vi "Windows Main-forDOG.vi"() -> ()   [LabVIEW 2016]
uses:
  <resource>/objmgr/ni.dex.rc
panel:
  in  "停止应用程序 15":bool
  out "Array 14":i32[][](array[numeric])
  in  "停止应用程序 14":bool
  out "Array 13":i32[][](array[numeric])
  in  "停止应用程序 13":bool
  out "Array 12":i32[][](array[numeric])
  in  "停止应用程序 12":bool
  out "Array 11":i32[][](array[numeric])
  in  "停止应用程序 11":bool
  out "Array 10":i32[][](array[numeric])
  in  "停止应用程序 10":bool
  out "Array 9":i32[][](array[numeric])
  in  "停止应用程序 9":bool
  out "Gaussian2-4":T1(plugin-control)
  out "Array 8":i32[][](array[numeric])
  in  "停止应用程序 8":bool
  out "Gaussian2-3":T1(plugin-control)
  out "Array 7":i32[][](array[numeric])
  in  "停止应用程序 7":bool
  out "Gaussian2-2":T1(plugin-control)
  out "Array 6":i32[][](array[numeric])
  in  "停止应用程序 6":bool
  out "Gaussian2-1":T1(plugin-control)
  out "Array 5":i32[][](array[numeric])
  in  "停止应用程序 5":bool
  out "Gaussian1-4":T1(plugin-control)
  out "Array 4":i32[][](array[numeric])
  in  "停止应用程序 4":bool
  out "Gaussian1-3":T1(plugin-control)
  out "Array 3":i32[][](array[numeric])
  in  "停止应用程序 3":bool
  out "Gaussian1-2":T1(plugin-control)
  out "Array 2":i32[][](array[numeric])
  out "error out 2":errorcluster
  in  "停止应用程序 2":bool
  out "OriImage":T1(plugin-control)
  out "Array":i32[][](array[numeric])
  out "Numeric":i32
  in  "终端IP地址":string
  out "error out":errorcluster
  in  "停止应用程序":bool
  out "Gaussian1-1":T1(plugin-control)
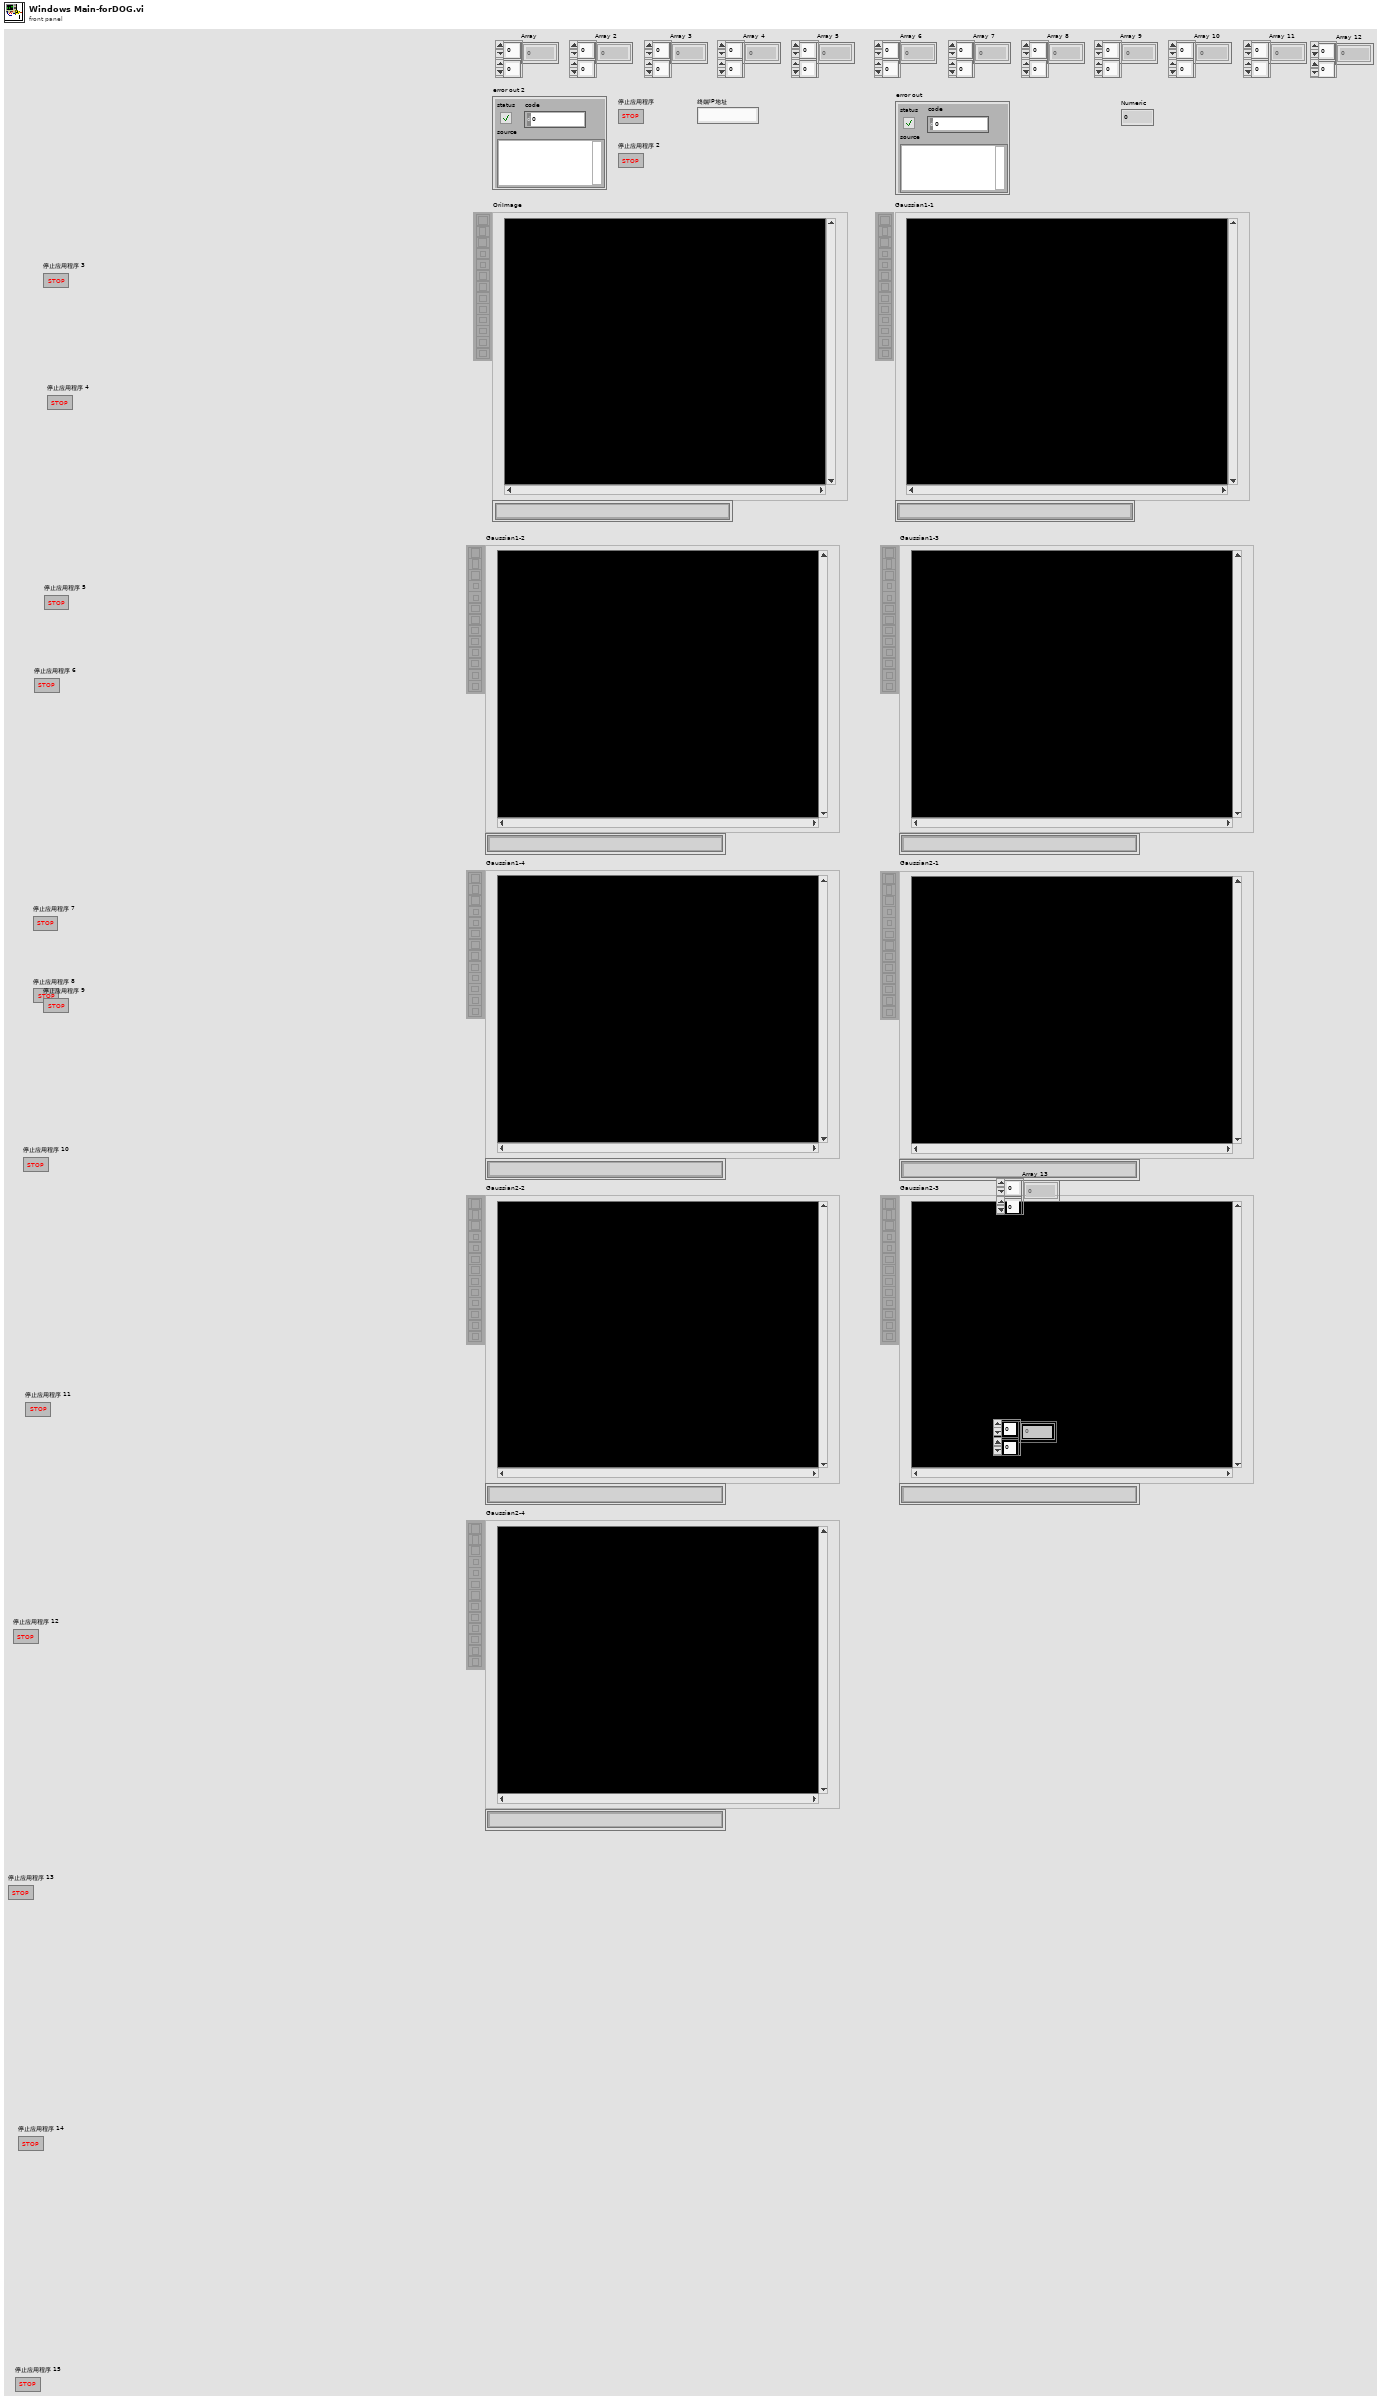
[diagram p1: front panel]
types:
  T1 = typedef "IMAQ Image.ctl" = refnum<image>
  T2 = typedef "Image Type" = u32
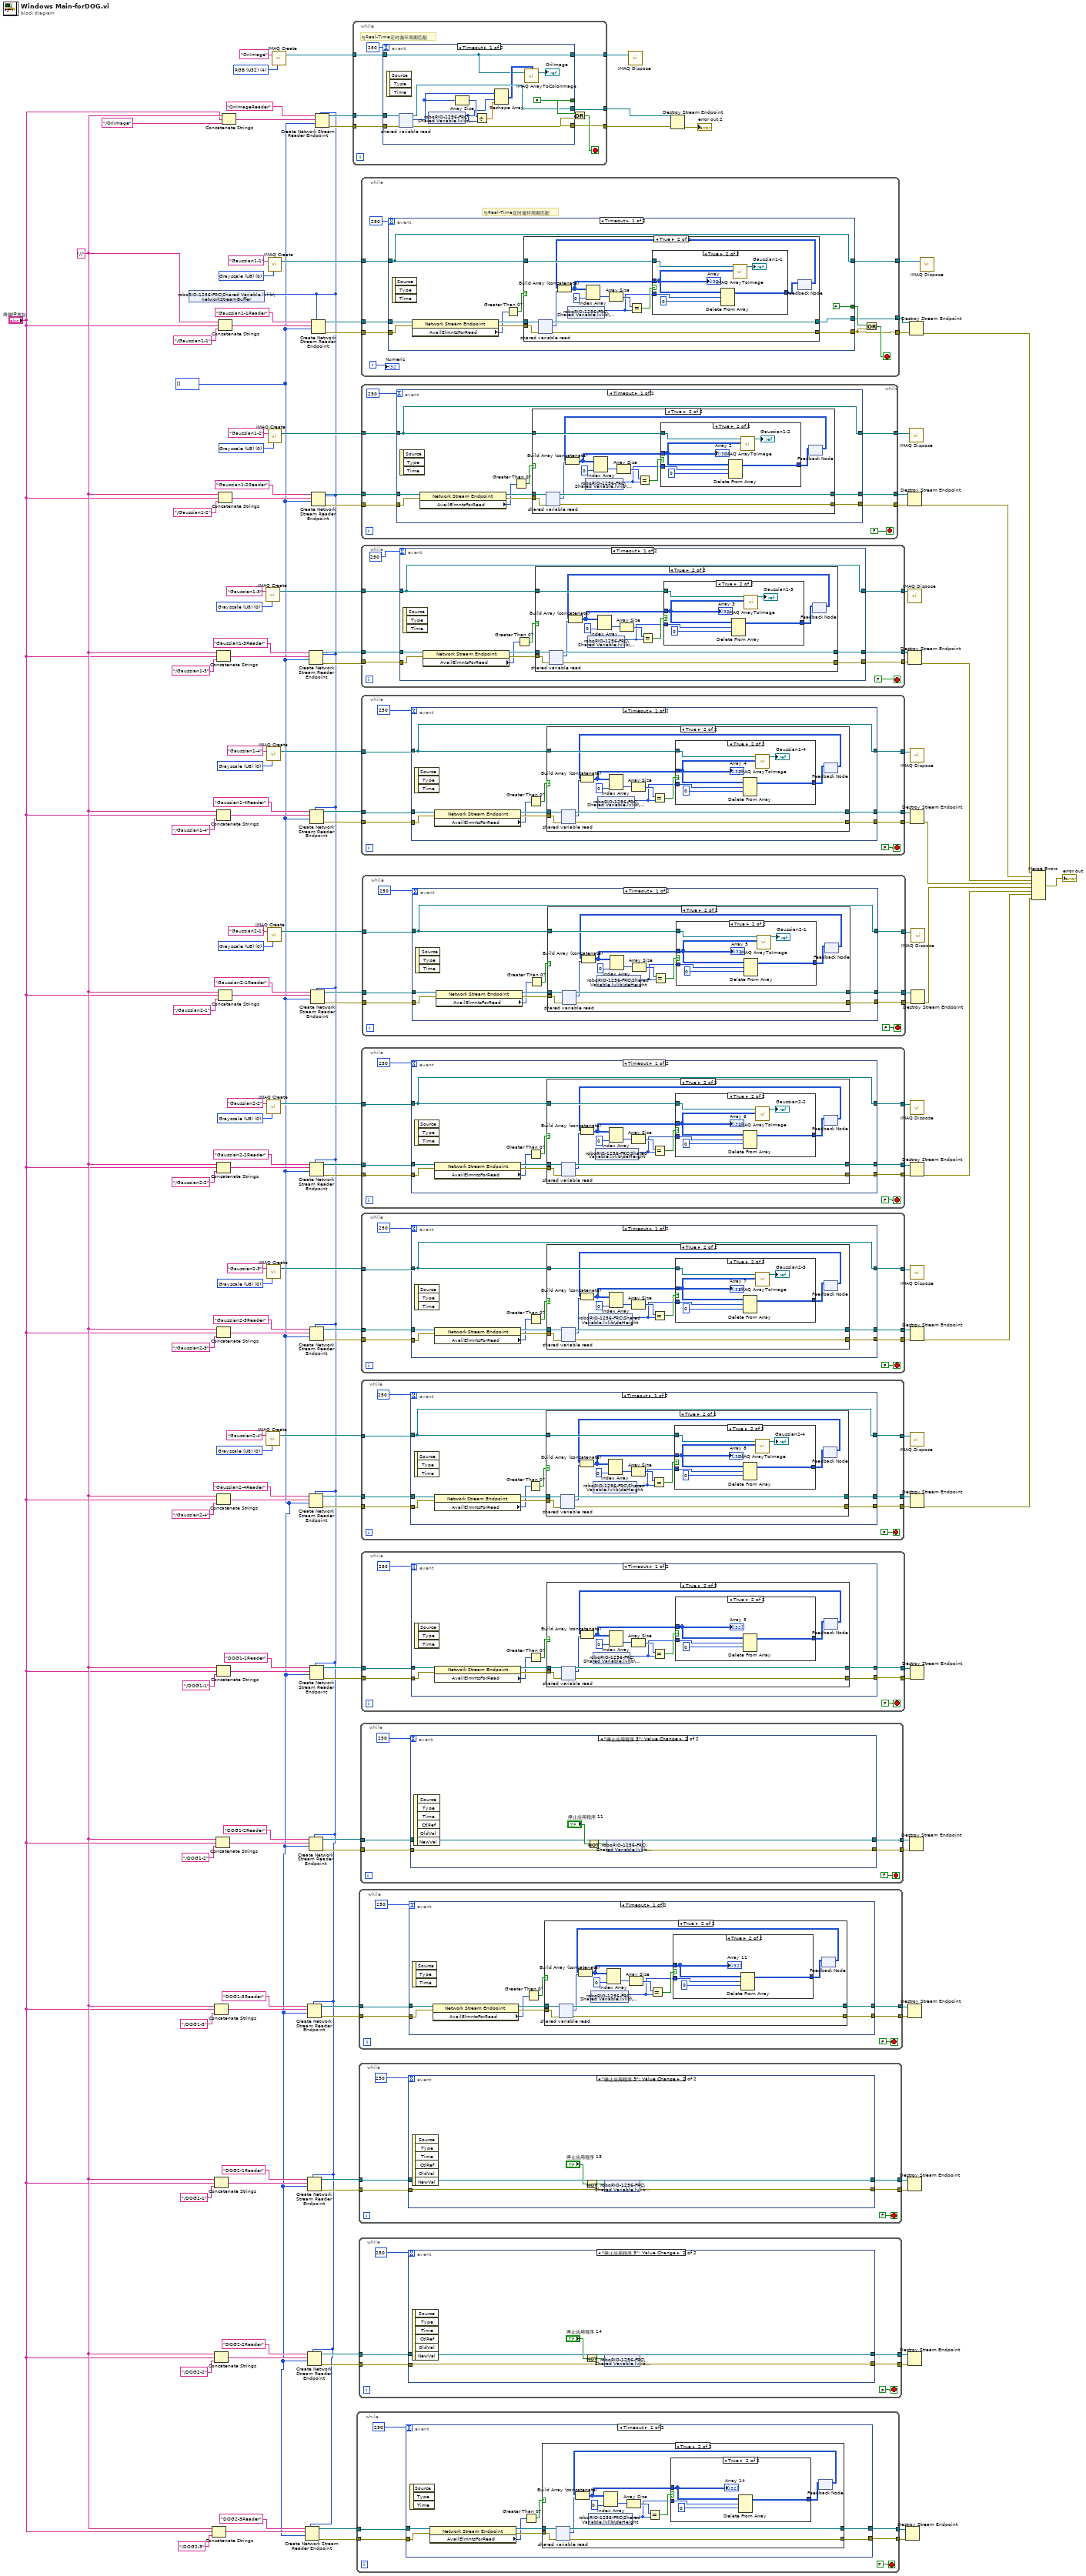
[diagram p0: block diagram]
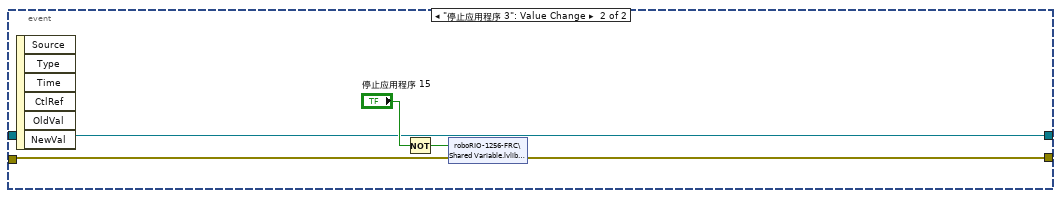
[diagram p4: hidden frame]
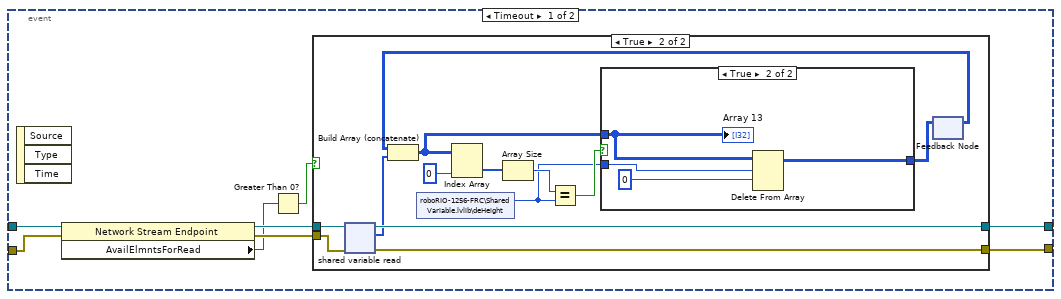
[diagram p5: hidden frame]
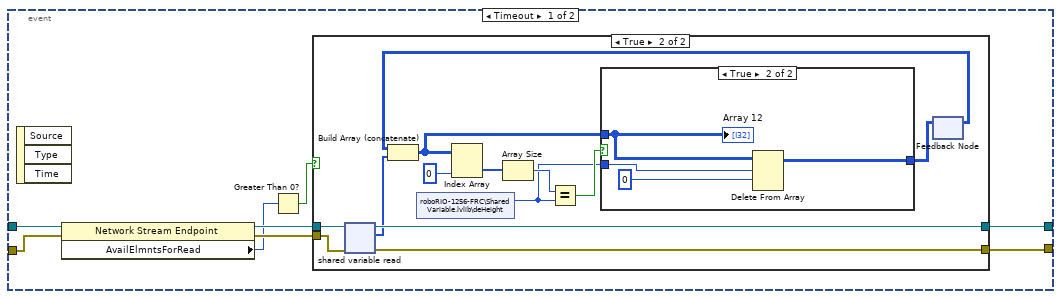
[diagram p8: hidden frame]
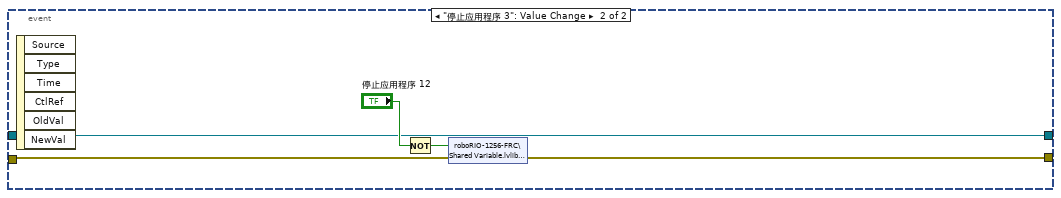
[diagram p13: hidden frame]
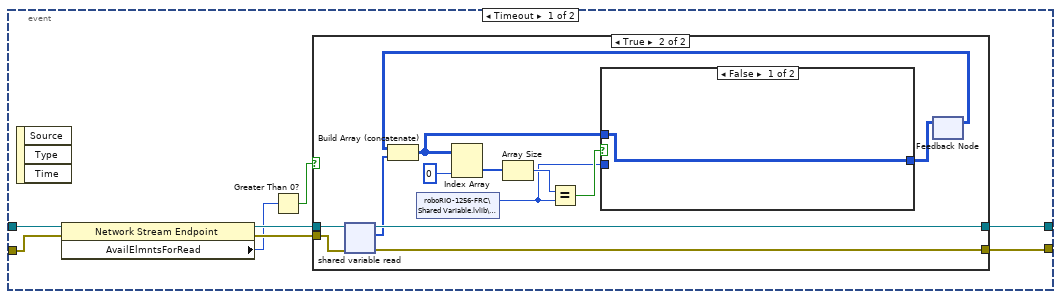
[diagram p14: hidden frame]
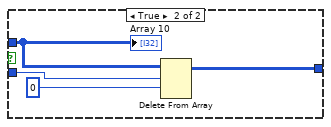
[diagram p16: hidden frame]
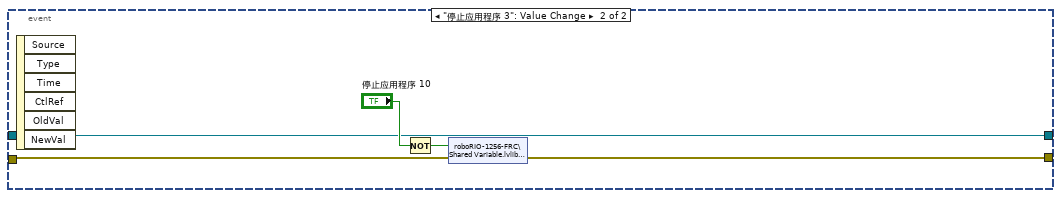
[diagram p19: hidden frame]
diagram:
  w60 = T2 0 items=["Grayscale (U8)", "Grayscale (I16)", "Grayscale (SGL)", "Complex (CSG)", "RGB (U32)", "HSL (U32)", "RGB (U64)", "Grayscale (U16)"] ("Image Type")
  w61 = T2 0 items=["Grayscale (U8)", "Grayscale (I16)", "Grayscale (SGL)", "Complex (CSG)", "RGB (U32)", "HSL (U32)", "RGB (U64)", "Grayscale (U16)"] ("Image Type")
  w82 = T2 0 items=["Grayscale (U8)", "Grayscale (I16)", "Grayscale (SGL)", "Complex (CSG)", "RGB (U32)", "HSL (U32)", "RGB (U64)", "Grayscale (U16)"] ("Image Type")
  w84 = T2 0 items=["Grayscale (U8)", "Grayscale (I16)", "Grayscale (SGL)", "Complex (CSG)", "RGB (U32)", "HSL (U32)", "RGB (U64)", "Grayscale (U16)"] ("Image Type")
  w118 = T2 0 items=["Grayscale (U8)", "Grayscale (I16)", "Grayscale (SGL)", "Complex (CSG)", "RGB (U32)", "HSL (U32)", "RGB (U64)", "Grayscale (U16)"] ("Image Type")
  w123 = T2 0 items=["Grayscale (U8)", "Grayscale (I16)", "Grayscale (SGL)", "Complex (CSG)", "RGB (U32)", "HSL (U32)", "RGB (U64)", "Grayscale (U16)"] ("Image Type")
  w124 = T2 0 items=["Grayscale (U8)", "Grayscale (I16)", "Grayscale (SGL)", "Complex (CSG)", "RGB (U32)", "HSL (U32)", "RGB (U64)", "Grayscale (U16)"] ("Image Type")
  w136 = T2 4 items=["Grayscale (U8)", "Grayscale (I16)", "Grayscale (SGL)", "Complex (CSG)", "RGB (U32)", "HSL (U32)", "RGB (U64)", "Grayscale (U16)"] ("Image Type")
  w129 = T2 0 items=["Grayscale (U8)", "Grayscale (I16)", "Grayscale (SGL)", "Complex (CSG)", "RGB (U32)", "HSL (U32)", "RGB (U64)", "Grayscale (U16)"] ("Image Type")
  w3 = i32[] []
  w2 = "//" ("string")
  n1 = shared-variable "roboRIO-1256-FRC\\Shared Variable.lvlib\\networkStreamBuffer"() -> (w4:i8)  [unwired: 1 in, 1 out]
  n2 = Concatenate Strings(w2, "终端IP地址", "/DOG2-3" ("string")) -> (w9:string)
  n3 = Concatenate Strings(w2, "终端IP地址", "/DOG2-1" ("string")) -> (w23:string)
  n4 = Concatenate Strings(w2, "终端IP地址", "/DOG2-2" ("string")) -> (w14:string)
  n5 = Concatenate Strings(w2, "终端IP地址", "/DOG1-3" ("string")) -> (w28:string)
  n6 = Concatenate Strings(w2, "终端IP地址", "/DOG1-2" ("string")) -> (w37:string)
  n7 = Concatenate Strings(w2, "终端IP地址", "/Gaussian1-3" ("string")) -> (w127:string)
  n8 = Concatenate Strings(w2, "终端IP地址", "/Gaussian2-4" ("string")) -> (w57:string)
  n9 = Concatenate Strings(w2, "终端IP地址", "/Gaussian1-4" ("string")) -> (w115:string)
  n10 = Concatenate Strings(w2, "终端IP地址", "/Gaussian2-2" ("string")) -> (w79:string)
  n11 = Concatenate Strings(w2, "终端IP地址", "/Gaussian2-3" ("string")) -> (w64:string)
  n12 = Concatenate Strings(w2, "终端IP地址", "/DOG1-1" ("string")) -> (w42:string)
  n13 = Concatenate Strings(w2, "终端IP地址", "/Gaussian2-1" ("string")) -> (w87:string)
  n14 = Concatenate Strings(w2, "终端IP地址", "/Gaussian1-1" ("string")) -> (w152:string)
  n15 = Concatenate Strings(w2, "终端IP地址", "/Gaussian1-2" ("string")) -> (w131:string)
  n16 = Concatenate Strings(w2, "终端IP地址", "/OriImage" ("string")) -> (w142:string)
  n17 = call "IMAQ Create"("Image Name"="Gaussian1-3", "Image Type"=w123) -> ("New Image"=w106:T1)  [unwired: 3 in, 1 out]
  n18 = call "IMAQ Create"("Image Name"="Gaussian2-4", "Image Type"=w60) -> ("New Image"=w55:T1)  [unwired: 3 in, 1 out]
  n19 = call "IMAQ Create"("Image Name"="Gaussian1-4", "Image Type"=w118) -> ("New Image"=w112:T1)  [unwired: 3 in, 1 out]
  n20 = call "IMAQ Create"("Image Name"="Gaussian2-2", "Image Type"=w82) -> ("New Image"=w77:T1)  [unwired: 3 in, 1 out]
  n21 = call "IMAQ Create"("Image Name"="Gaussian2-3", "Image Type"=w61) -> ("New Image"=w66:T1)  [unwired: 3 in, 1 out]
  n22 = call "IMAQ Create"("Image Name"="Gaussian2-1", "Image Type"=w84) -> ("New Image"=w89:T1)  [unwired: 3 in, 1 out]
  n23 = call "IMAQ Create"("Image Name"="Gaussian1-1", "Image Type"=w129) -> ("New Image"=w148:T1)  [unwired: 3 in, 1 out]
  n24 = call "IMAQ Create"("Image Name"="Gaussian1-2", "Image Type"=w124) -> ("New Image"=w98:T1)  [unwired: 3 in, 1 out]
  n25 = call "IMAQ Create"("Image Name"="OriImage", "Image Type"=w136) -> ("New Image"=w135:T1)  [unwired: 3 in, 1 out]
  n26 = Create Network Stream Reader Endpoint(7:w4, 9:w3, 10:w9, 11:"DOG2-3Reader" ("reader name")) -> (0:w7:errorcluster, 3:w8:refnum<k21>)  [unwired: 3 in]
  n27 = Create Network Stream Reader Endpoint(7:w4, 9:w3, 10:w23, 11:"DOG2-1Reader" ("reader name")) -> (0:w21:errorcluster, 3:w22:refnum<k21>)  [unwired: 3 in]
  n28 = Create Network Stream Reader Endpoint(7:w4, 9:w3, 10:w14, 11:"DOG2-2Reader" ("reader name")) -> (0:w16:errorcluster, 3:w15:refnum<k21>)  [unwired: 3 in]
  n29 = Create Network Stream Reader Endpoint(7:w4, 9:w3, 10:w28, 11:"DOG1-3Reader" ("reader name")) -> (0:w30:errorcluster, 3:w29:refnum<k21>)  [unwired: 3 in]
  n30 = Create Network Stream Reader Endpoint(7:w4, 9:w3, 10:w37, 11:"DOG1-2Reader" ("reader name")) -> (0:w35:errorcluster, 3:w36:refnum<k21>)  [unwired: 3 in]
  n31 = Create Network Stream Reader Endpoint(7:w4, 9:w3, 10:w127, 11:"Gaussian1-3Reader" ("reader name")) -> (0:w104:errorcluster, 3:w105:refnum<k21>)  [unwired: 3 in]
  n32 = Create Network Stream Reader Endpoint(7:w4, 9:w3, 10:w57, 11:"Gaussian2-4Reader" ("reader name")) -> (0:w53:errorcluster, 3:w54:refnum<k21>)  [unwired: 3 in]
  n33 = Create Network Stream Reader Endpoint(7:w4, 9:w3, 10:w115, 11:"Gaussian1-4Reader" ("reader name")) -> (0:w110:errorcluster, 3:w111:refnum<k21>)  [unwired: 3 in]
  n34 = Create Network Stream Reader Endpoint(7:w4, 9:w3, 10:w79, 11:"Gaussian2-2Reader" ("reader name")) -> (0:w75:errorcluster, 3:w76:refnum<k21>)  [unwired: 3 in]
  n35 = Create Network Stream Reader Endpoint(7:w4, 9:w3, 10:w64, 11:"Gaussian2-3Reader" ("reader name")) -> (0:w68:errorcluster, 3:w67:refnum<k21>)  [unwired: 3 in]
  n36 = Create Network Stream Reader Endpoint(7:w4, 9:w3, 10:w42, 11:"DOG1-1Reader" ("reader name")) -> (0:w44:errorcluster, 3:w43:refnum<k21>)  [unwired: 3 in]
  n37 = Create Network Stream Reader Endpoint(7:w4, 9:w3, 10:w87, 11:"Gaussian2-1Reader" ("reader name")) -> (0:w91:errorcluster, 3:w90:refnum<k21>)  [unwired: 3 in]
  n38 = Create Network Stream Reader Endpoint(7:w4, 9:w3, 10:w152, 11:"Gaussian1-1Reader" ("reader name")) -> (0:w155:errorcluster, 3:w146:refnum<k21>)  [unwired: 3 in]
  n39 = Create Network Stream Reader Endpoint(7:w4, 9:w3, 10:w131, 11:"Gaussian1-2Reader" ("reader name")) -> (0:w99:errorcluster, 3:w100:refnum<k21>)  [unwired: 3 in]
  n40 = Create Network Stream Reader Endpoint(7:w4, 9:w3, 10:w142, 11:"OriImageReader" ("reader name")) -> (0:w145:errorcluster, 3:w140:refnum<k21>)  [unwired: 3 in]
  n41 = while {
    tunnel: w140 -> [w159]
    tunnel: [w158] -> w139
    tunnel: w135 -> [w157]
    tunnel: [w156] -> w134
    tunnel: w145 -> [w161]
    tunnel: [w160] -> w141
    stop <- w162 stop-if-true
    # "与Real-Time定时循环周期匹配"
    n42 = event shown="[0] Timeout" {
      selector: _ -> [_ _]
      dyn-events: _ -> [_ _]
      timeout: 250 -> [_ _]
      tunnel: [FALSE ("停止应用程序") "停止应用程序 2"] -> w163
      tunnel: w161 -> [w176 w180]
      tunnel: [w175 w179] -> w160
      tunnel: w159 -> [w174 w177]
      tunnel: [w173 w177] -> w158
      tunnel: w157 -> [w166 w178]
      tunnel: [w166 w178] -> w156
      event Timeout {
        n43 = event-data() -> ()  [unwired: 1 in, 3 out]
        n44 = shared-variable-read(w174, w176) -> (w173:refnum<k21>, w175:errorcluster, w169:i32[])  [unwired: 1 in, 1 out]
        n45 = shared-variable "roboRIO-1256-FRC\\Shared Variable.lvlib\\Height"() -> (w165:u16)  [unwired: 1 in, 1 out]
        n46 = Array Size(array=w169) -> (size(s)=w171:i32)
        n47 = Divide(x=w171, y=w165) -> (x/y=w170:dbl)
        n48 = Reshape Array(w169, w165, w170) -> (w168:i32[][])
        n49 = call "IMAQ ArrayToColorImage"("Image Pixels (U32)"=w168, "Image"=w166) -> ("Image Out"=→"OriImage":T1)  [unwired: 3 in, 1 out]
      }
      event "停止应用程序 2": Value Change {
        n50 = event-data() -> ()  [unwired: 1 in, 6 out]
        n51 = Not(x="停止应用程序 2") -> (.not. x?=w181:bool)
        n52 = shared-variable "roboRIO-1256-FRC\\Shared Variable.lvlib\\Active"(w181, error in=w180) -> (error out=w179:errorcluster)
      }
    }
    n53 = Or(x=w163, y=w160) -> (x .or. y?=w162:bool)
  }
  n54 = while {
    tunnel: w8 -> [w188]
    tunnel: [w185] -> w5
    tunnel: w7 -> [w187]
    tunnel: [w186] -> w6
    stop <- FALSE stop-if-true
    n55 = event shown="[0] Timeout" {
      selector: _ -> [_ _]
      dyn-events: _ -> [_ _]
      timeout: 250 -> [_ _]
      tunnel: w187 -> [w194 w219]
      tunnel: [w196 w218] -> w186
      tunnel: w188 -> [w193 w217]
      tunnel: [w195 w217] -> w185
      event Timeout {
        n56 = event-data() -> ()  [unwired: 1 in, 3 out]
        n57 = property class="Network Stream Endpoint"(reference=w193, error in=w194) -> (reference out=w191:refnum<k21>, error out=w192:errorcluster, "AvailElmntsForRead"=w190:i32)
        n58 = Greater Than 0?(x=w190) -> (x > 0?=w189:bool)
        n59 = case shown="True" w189 {
          tunnel: [w197 w211] -> w196
          tunnel: [w198 w210] -> w195
          tunnel: w192 -> [w197 w205]
          tunnel: w191 -> [w198 w204]
          frame False {
          }
          frame True {
            n60 = shared-variable-read(w204, w205) -> (w210:refnum<k21>, w211:errorcluster, w202:i32[])  [unwired: 1 in, 1 out]
            n61 = shared-variable "roboRIO-1256-FRC\\Shared Variable.lvlib\\deHeight"() -> (w199:u16)  [unwired: 1 in, 1 out]
            n62 = feedback #1() -> (w200:i32[][])  [unwired: 1 in]
            n63 = Build Array (concatenate)(w200, w202) -> (w203:i32[][])
            n64 = Index Array(array=w203, index (col)=0 ("disabled index (col)")) -> (element=w208:i32[])  [unwired: 1 in]
            n65 = Array Size(array=w208) -> (size(s)=w207:i32)
            n66 = Equal?(x=w207, y=w199) -> (x = y?=w206:bool)
            n67 = case shown="True" w206 {
              tunnel: w203 -> [w212 w213]
              tunnel: [w212 w214] -> w201
              tunnel: w199 -> [_ w216]
              frame False {
              }
              frame True {
                n68 = Delete From Array(array=w213, length=w216, index (row)=0) -> (array with subset deleted=w214:i32[][])  [unwired: 1 in, 1 out]
                "Array 14" <- w213
              }
            }
            n69 = feedback-in #1(w201) -> ()
          }
        }
      }
      event "停止应用程序 3": Value Change {
        n70 = event-data() -> ()  [unwired: 1 in, 6 out]
        n71 = Not(x="停止应用程序 15") -> (.not. x?=w220:bool)
        n72 = shared-variable "roboRIO-1256-FRC\\Shared Variable.lvlib\\Active"(w220, error in=w219) -> (error out=w218:errorcluster)
      }
    }
  }
  n73 = while {
    tunnel: w22 -> [w227]
    tunnel: [w224] -> w19
    tunnel: w21 -> [w226]
    tunnel: [w225] -> w20
    stop <- FALSE stop-if-true
    n74 = event shown="[1] \"停止应用程序 3\": Value Change" {
      selector: _ -> [_ _]
      dyn-events: _ -> [_ _]
      timeout: 250 -> [_ _]
      tunnel: w226 -> [w233 w258]
      tunnel: [w235 w257] -> w225
      tunnel: w227 -> [w232 w256]
      tunnel: [w234 w256] -> w224
      event Timeout {
        n75 = event-data() -> ()  [unwired: 1 in, 3 out]
        n76 = property class="Network Stream Endpoint"(reference=w232, error in=w233) -> (reference out=w230:refnum<k21>, error out=w231:errorcluster, "AvailElmntsForRead"=w229:i32)
        n77 = Greater Than 0?(x=w229) -> (x > 0?=w228:bool)
        n78 = case shown="True" w228 {
          tunnel: [w236 w250] -> w235
          tunnel: [w237 w249] -> w234
          tunnel: w231 -> [w236 w244]
          tunnel: w230 -> [w237 w243]
          frame False {
          }
          frame True {
            n79 = shared-variable-read(w243, w244) -> (w249:refnum<k21>, w250:errorcluster, w241:i32[])  [unwired: 1 in, 1 out]
            n80 = shared-variable "roboRIO-1256-FRC\\Shared Variable.lvlib\\deHeight"() -> (w238:u16)  [unwired: 1 in, 1 out]
            n81 = feedback #2() -> (w239:i32[][])  [unwired: 1 in]
            n82 = Build Array (concatenate)(w239, w241) -> (w242:i32[][])
            n83 = Index Array(array=w242, index (col)=0 ("disabled index (col)")) -> (element=w247:i32[])  [unwired: 1 in]
            n84 = Array Size(array=w247) -> (size(s)=w246:i32)
            n85 = Equal?(x=w246, y=w238) -> (x = y?=w245:bool)
            n86 = case shown="True" w245 {
              tunnel: w242 -> [w251 w252]
              tunnel: [w251 w253] -> w240
              tunnel: w238 -> [_ w255]
              frame False {
              }
              frame True {
                n87 = Delete From Array(array=w252, length=w255, index (row)=0) -> (array with subset deleted=w253:i32[][])  [unwired: 1 in, 1 out]
                "Array 12" <- w252
              }
            }
            n88 = feedback-in #2(w240) -> ()
          }
        }
      }
      event "停止应用程序 3": Value Change {
        n89 = event-data() -> ()  [unwired: 1 in, 6 out]
        n90 = Not(x="停止应用程序 13") -> (.not. x?=w259:bool)
        n91 = shared-variable "roboRIO-1256-FRC\\Shared Variable.lvlib\\Active"(w259, error in=w258) -> (error out=w257:errorcluster)
      }
    }
  }
  n92 = while {
    tunnel: w15 -> [w266]
    tunnel: [w263] -> w18
    tunnel: w16 -> [w265]
    tunnel: [w264] -> w17
    stop <- FALSE stop-if-true
    n93 = event shown="[1] \"停止应用程序 3\": Value Change" {
      selector: _ -> [_ _]
      dyn-events: _ -> [_ _]
      timeout: 250 -> [_ _]
      tunnel: w265 -> [w272 w297]
      tunnel: [w274 w296] -> w264
      tunnel: w266 -> [w271 w295]
      tunnel: [w273 w295] -> w263
      event Timeout {
        n94 = event-data() -> ()  [unwired: 1 in, 3 out]
        n95 = property class="Network Stream Endpoint"(reference=w271, error in=w272) -> (reference out=w269:refnum<k21>, error out=w270:errorcluster, "AvailElmntsForRead"=w268:i32)
        n96 = Greater Than 0?(x=w268) -> (x > 0?=w267:bool)
        n97 = case shown="True" w267 {
          tunnel: [w275 w289] -> w274
          tunnel: [w276 w288] -> w273
          tunnel: w270 -> [w275 w283]
          tunnel: w269 -> [w276 w282]
          frame False {
          }
          frame True {
            n98 = shared-variable-read(w282, w283) -> (w288:refnum<k21>, w289:errorcluster, w280:i32[])  [unwired: 1 in, 1 out]
            n99 = shared-variable "roboRIO-1256-FRC\\Shared Variable.lvlib\\deHeight"() -> (w277:u16)  [unwired: 1 in, 1 out]
            n100 = feedback #3() -> (w278:i32[][])  [unwired: 1 in]
            n101 = Build Array (concatenate)(w278, w280) -> (w281:i32[][])
            n102 = Index Array(array=w281, index (col)=0 ("disabled index (col)")) -> (element=w286:i32[])  [unwired: 1 in]
            n103 = Array Size(array=w286) -> (size(s)=w285:i32)
            n104 = Equal?(x=w285, y=w277) -> (x = y?=w284:bool)
            n105 = case shown="True" w284 {
              tunnel: w281 -> [w290 w291]
              tunnel: [w290 w292] -> w279
              tunnel: w277 -> [_ w294]
              frame False {
              }
              frame True {
                n106 = Delete From Array(array=w291, length=w294, index (row)=0) -> (array with subset deleted=w292:i32[][])  [unwired: 1 in, 1 out]
                "Array 13" <- w291
              }
            }
            n107 = feedback-in #3(w279) -> ()
          }
        }
      }
      event "停止应用程序 3": Value Change {
        n108 = event-data() -> ()  [unwired: 1 in, 6 out]
        n109 = Not(x="停止应用程序 14") -> (.not. x?=w298:bool)
        n110 = shared-variable "roboRIO-1256-FRC\\Shared Variable.lvlib\\Active"(w298, error in=w297) -> (error out=w296:errorcluster)
      }
    }
  }
  n111 = while {
    tunnel: w29 -> [w305]
    tunnel: [w302] -> w32
    tunnel: w30 -> [w304]
    tunnel: [w303] -> w31
    stop <- FALSE stop-if-true
    n112 = event shown="[0] Timeout" {
      selector: _ -> [_ _]
      dyn-events: _ -> [_ _]
      timeout: 250 -> [_ _]
      tunnel: w304 -> [w311 w336]
      tunnel: [w313 w335] -> w303
      tunnel: w305 -> [w310 w334]
      tunnel: [w312 w334] -> w302
      event Timeout {
        n113 = event-data() -> ()  [unwired: 1 in, 3 out]
        n114 = property class="Network Stream Endpoint"(reference=w310, error in=w311) -> (reference out=w308:refnum<k21>, error out=w309:errorcluster, "AvailElmntsForRead"=w307:i32)
        n115 = Greater Than 0?(x=w307) -> (x > 0?=w306:bool)
        n116 = case shown="True" w306 {
          tunnel: [w314 w328] -> w313
          tunnel: [w315 w327] -> w312
          tunnel: w309 -> [w314 w322]
          tunnel: w308 -> [w315 w321]
          frame False {
          }
          frame True {
            n117 = shared-variable-read(w321, w322) -> (w327:refnum<k21>, w328:errorcluster, w319:i32[])  [unwired: 1 in, 1 out]
            n118 = shared-variable "roboRIO-1256-FRC\\Shared Variable.lvlib\\Height"() -> (w316:u16)  [unwired: 1 in, 1 out]
            n119 = feedback #4() -> (w317:i32[][])  [unwired: 1 in]
            n120 = Build Array (concatenate)(w317, w319) -> (w320:i32[][])
            n121 = Index Array(array=w320, index (col)=0 ("disabled index (col)")) -> (element=w325:i32[])  [unwired: 1 in]
            n122 = Array Size(array=w325) -> (size(s)=w324:i32)
            n123 = Equal?(x=w324, y=w316) -> (x = y?=w323:bool)
            n124 = case shown="True" w323 {
              tunnel: w320 -> [w329 w330]
              tunnel: [w329 w331] -> w318
              tunnel: w316 -> [_ w333]
              frame False {
              }
              frame True {
                n125 = Delete From Array(array=w330, length=w333, index (row)=0) -> (array with subset deleted=w331:i32[][])  [unwired: 1 in, 1 out]
                "Array 11" <- w330
              }
            }
            n126 = feedback-in #4(w318) -> ()
          }
        }
      }
      event "停止应用程序 3": Value Change {
        n127 = event-data() -> ()  [unwired: 1 in, 6 out]
        n128 = Not(x="停止应用程序 12") -> (.not. x?=w337:bool)
        n129 = shared-variable "roboRIO-1256-FRC\\Shared Variable.lvlib\\Active"(w337, error in=w336) -> (error out=w335:errorcluster)
      }
    }
  }
  n130 = while {
    tunnel: w36 -> [w344]
    tunnel: [w341] -> w33
    tunnel: w35 -> [w343]
    tunnel: [w342] -> w34
    stop <- FALSE stop-if-true
    n131 = event shown="[1] \"停止应用程序 3\": Value Change" {
      selector: _ -> [_ _]
      dyn-events: _ -> [_ _]
      timeout: 250 -> [_ _]
      tunnel: w343 -> [w350 w375]
      tunnel: [w352 w374] -> w342
      tunnel: w344 -> [w349 w373]
      tunnel: [w351 w373] -> w341
      event Timeout {
        n132 = event-data() -> ()  [unwired: 1 in, 3 out]
        n133 = property class="Network Stream Endpoint"(reference=w349, error in=w350) -> (reference out=w347:refnum<k21>, error out=w348:errorcluster, "AvailElmntsForRead"=w346:i32)
        n134 = Greater Than 0?(x=w346) -> (x > 0?=w345:bool)
        n135 = case shown="True" w345 {
          tunnel: [w353 w367] -> w352
          tunnel: [w354 w366] -> w351
          tunnel: w348 -> [w353 w361]
          tunnel: w347 -> [w354 w360]
          frame False {
          }
          frame True {
            n136 = shared-variable-read(w360, w361) -> (w366:refnum<k21>, w367:errorcluster, w358:i32[])  [unwired: 1 in, 1 out]
            n137 = shared-variable "roboRIO-1256-FRC\\Shared Variable.lvlib\\Height"() -> (w355:u16)  [unwired: 1 in, 1 out]
            n138 = feedback #5() -> (w356:i32[][])  [unwired: 1 in]
            n139 = Build Array (concatenate)(w356, w358) -> (w359:i32[][])
            n140 = Index Array(array=w359, index (col)=0 ("disabled index (col)")) -> (element=w364:i32[])  [unwired: 1 in]
            n141 = Array Size(array=w364) -> (size(s)=w363:i32)
            n142 = Equal?(x=w363, y=w355) -> (x = y?=w362:bool)
            n143 = case shown="False" w362 {
              tunnel: w359 -> [w368 w369]
              tunnel: [w368 w370] -> w357
              tunnel: w355 -> [_ w372]
              frame False {
              }
              frame True {
                n144 = Delete From Array(array=w369, length=w372, index (row)=0) -> (array with subset deleted=w370:i32[][])  [unwired: 1 in, 1 out]
                "Array 10" <- w369
              }
            }
            n145 = feedback-in #5(w357) -> ()
          }
        }
      }
      event "停止应用程序 3": Value Change {
        n146 = event-data() -> ()  [unwired: 1 in, 6 out]
        n147 = Not(x="停止应用程序 11") -> (.not. x?=w376:bool)
        n148 = shared-variable "roboRIO-1256-FRC\\Shared Variable.lvlib\\Active"(w376, error in=w375) -> (error out=w374:errorcluster)
      }
    }
  }
  n149 = while {
    tunnel: w55 -> [w385]
    tunnel: [w380] -> w50
    tunnel: w54 -> [w384]
    tunnel: [w381] -> w51
    tunnel: w53 -> [w383]
    tunnel: [w382] -> w52
    stop <- FALSE stop-if-true
    n150 = event shown="[0] Timeout" {
      selector: _ -> [_ _]
      dyn-events: _ -> [_ _]
      timeout: 250 -> [_ _]
      tunnel: w383 -> [w391 w421]
      tunnel: [w394 w420] -> w382
      tunnel: w384 -> [w390 w418]
      tunnel: [w393 w418] -> w381
      tunnel: w385 -> [w392 w419]
      tunnel: [w392 w419] -> w380
      event Timeout {
        n151 = event-data() -> ()  [unwired: 1 in, 3 out]
        n152 = property class="Network Stream Endpoint"(reference=w390, error in=w391) -> (reference out=w388:refnum<k21>, error out=w389:errorcluster, "AvailElmntsForRead"=w387:i32)
        n153 = Greater Than 0?(x=w387) -> (x > 0?=w386:bool)
        n154 = case shown="True" w386 {
          tunnel: [w395 w410] -> w394
          tunnel: [w396 w409] -> w393
          tunnel: w392 -> [_ w402]
          tunnel: w389 -> [w395 w404]
          tunnel: w388 -> [w396 w403]
          frame False {
          }
          frame True {
            n155 = shared-variable-read(w403, w404) -> (w409:refnum<k21>, w410:errorcluster, w400:i32[])  [unwired: 1 in, 1 out]
            n156 = shared-variable "roboRIO-1256-FRC\\Shared Variable.lvlib\\deHeight"() -> (w397:u16)  [unwired: 1 in, 1 out]
            n157 = feedback #6() -> (w398:i32[][])  [unwired: 1 in]
            n158 = Build Array (concatenate)(w398, w400) -> (w401:i32[][])
            n159 = Index Array(array=w401, index (col)=0 ("disabled index (col)")) -> (element=w407:i32[])  [unwired: 1 in]
            n160 = Array Size(array=w407) -> (size(s)=w406:i32)
            n161 = Equal?(x=w406, y=w397) -> (x = y?=w405:bool)
            n162 = case shown="True" w405 {
              tunnel: w401 -> [w411 w412]
              tunnel: [w411 w413] -> w399
              tunnel: w397 -> [_ w417]
              tunnel: w402 -> [_ w414]
              frame False {
              }
              frame True {
                n163 = Delete From Array(array=w412, length=w417, index (row)=0) -> (array with subset deleted=w413:i32[][])  [unwired: 1 in, 1 out]
                n164 = call "IMAQ ArrayToImage"("Image Pixels (U8)"=w412, "Image"=w414) -> ("Image Out"=→"Gaussian2-4":T1)  [unwired: 8 in, 1 out]
                "Array 8" <- w412
              }
            }
            n165 = feedback-in #6(w399) -> ()
          }
        }
      }
      event "停止应用程序 3": Value Change {
        n166 = event-data() -> ()  [unwired: 1 in, 6 out]
        n167 = Not(x="停止应用程序 9") -> (.not. x?=w422:bool)
        n168 = shared-variable "roboRIO-1256-FRC\\Shared Variable.lvlib\\Active"(w422, error in=w421) -> (error out=w420:errorcluster)
      }
    }
  }
  n169 = while {
    tunnel: w146 -> [w428]
    tunnel: [w427] -> w150
    tunnel: w148 -> [w426]
    tunnel: [w425] -> w147
    tunnel: w155 -> [w430]
    tunnel: [w429] -> w151
    i -> [w424]
    stop <- w431 stop-if-true
    # "与Real-Time定时循环周期匹配"
    n170 = event shown="[0] Timeout" {
      selector: _ -> [_ _]
      dyn-events: _ -> [_ _]
      timeout: 250 -> [_ _]
      tunnel: [FALSE ("停止应用程序") "停止应用程序"] -> w432
      tunnel: w430 -> [w439 w470]
      tunnel: [w443 w469] -> w429
      tunnel: w428 -> [w438 w467]
      tunnel: [w442 w467] -> w427
      tunnel: w426 -> [w440 w468]
      tunnel: [w440 w468] -> w425
      event Timeout {
        n171 = event-data() -> ()  [unwired: 1 in, 3 out]
        n172 = property class="Network Stream Endpoint"(reference=w438, error in=w439) -> (reference out=w436:refnum<k21>, error out=w437:errorcluster, "AvailElmntsForRead"=w435:i32)
        n173 = Greater Than 0?(x=w435) -> (x > 0?=w434:bool)
        n174 = case shown="True" w434 {
          tunnel: [w444 w459] -> w443
          tunnel: [w445 w458] -> w442
          tunnel: w440 -> [_ w451]
          tunnel: w437 -> [w444 w453]
          tunnel: w436 -> [w445 w452]
          frame False {
          }
          frame True {
            n175 = shared-variable-read(w452, w453) -> (w458:refnum<k21>, w459:errorcluster, w449:i32[])  [unwired: 1 in, 1 out]
            n176 = shared-variable "roboRIO-1256-FRC\\Shared Variable.lvlib\\Height"() -> (w446:u16)  [unwired: 1 in, 1 out]
            n177 = feedback #7() -> (w447:i32[][])  [unwired: 1 in]
            n178 = Build Array (concatenate)(w447, w449) -> (w450:i32[][])
            n179 = Index Array(array=w450, index (col)=0 ("disabled index (col)")) -> (element=w456:i32[])  [unwired: 1 in]
            n180 = Array Size(array=w456) -> (size(s)=w455:i32)
            n181 = Equal?(x=w455, y=w446) -> (x = y?=w454:bool)
            n182 = case shown="True" w454 {
              tunnel: w450 -> [w460 w461]
              tunnel: [w460 w462] -> w448
              tunnel: w446 -> [_ w466]
              tunnel: w451 -> [_ w463]
              frame False {
              }
              frame True {
                n183 = Delete From Array(array=w461, length=w466, index (row)=0) -> (array with subset deleted=w462:i32[][])  [unwired: 1 in, 1 out]
                n184 = call "IMAQ ArrayToImage"("Image Pixels (U8)"=w461, "Image"=w463) -> ("Image Out"=→"Gaussian1-1":T1)  [unwired: 8 in, 1 out]
                "Array" <- w461
              }
            }
            n185 = feedback-in #7(w448) -> ()
          }
        }
      }
      event "停止应用程序": Value Change {
        n186 = event-data() -> ()  [unwired: 1 in, 6 out]
        n187 = Not(x="停止应用程序") -> (.not. x?=w471:bool)
        n188 = shared-variable "roboRIO-1256-FRC\\Shared Variable.lvlib\\Active"(w471, error in=w470) -> (error out=w469:errorcluster)
      }
    }
    n189 = Or(x=w432, y=w429) -> (x .or. y?=w431:bool)
    "Numeric" <- w424
  }
  n190 = while {
    tunnel: w98 -> [w478]
    tunnel: [w477] -> w97
    tunnel: w100 -> [w480]
    tunnel: [w476] -> w96
    tunnel: w99 -> [w479]
    tunnel: [w475] -> w95
    stop <- FALSE stop-if-true
    n191 = event shown="[0] Timeout" {
      selector: _ -> [_ _]
      dyn-events: _ -> [_ _]
      timeout: 250 -> [_ _]
      tunnel: w479 -> [w486 w516]
      tunnel: [w489 w515] -> w475
      tunnel: w480 -> [w485 w513]
      tunnel: [w488 w513] -> w476
      tunnel: w478 -> [w487 w514]
      tunnel: [w487 w514] -> w477
      event Timeout {
        n192 = event-data() -> ()  [unwired: 1 in, 3 out]
        n193 = property class="Network Stream Endpoint"(reference=w485, error in=w486) -> (reference out=w483:refnum<k21>, error out=w484:errorcluster, "AvailElmntsForRead"=w482:i32)
        n194 = Greater Than 0?(x=w482) -> (x > 0?=w481:bool)
        n195 = case shown="True" w481 {
          tunnel: [w490 w505] -> w489
          tunnel: [w491 w504] -> w488
          tunnel: w487 -> [_ w497]
          tunnel: w484 -> [w490 w499]
          tunnel: w483 -> [w491 w498]
          frame False {
          }
          frame True {
            n196 = shared-variable-read(w498, w499) -> (w504:refnum<k21>, w505:errorcluster, w495:i32[])  [unwired: 1 in, 1 out]
            n197 = shared-variable "roboRIO-1256-FRC\\Shared Variable.lvlib\\Height"() -> (w492:u16)  [unwired: 1 in, 1 out]
            n198 = feedback #8() -> (w493:i32[][])  [unwired: 1 in]
            n199 = Build Array (concatenate)(w493, w495) -> (w496:i32[][])
            n200 = Index Array(array=w496, index (col)=0 ("disabled index (col)")) -> (element=w502:i32[])  [unwired: 1 in]
            n201 = Array Size(array=w502) -> (size(s)=w501:i32)
            n202 = Equal?(x=w501, y=w492) -> (x = y?=w500:bool)
            n203 = case shown="True" w500 {
              tunnel: w496 -> [w506 w507]
              tunnel: [w506 w508] -> w494
              tunnel: w492 -> [_ w512]
              tunnel: w497 -> [_ w509]
              frame False {
              }
              frame True {
                n204 = Delete From Array(array=w507, length=w512, index (row)=0) -> (array with subset deleted=w508:i32[][])  [unwired: 1 in, 1 out]
                n205 = call "IMAQ ArrayToImage"("Image Pixels (U8)"=w507, "Image"=w509) -> ("Image Out"=→"Gaussian1-2":T1)  [unwired: 8 in, 1 out]
                "Array 2" <- w507
              }
            }
            n206 = feedback-in #8(w494) -> ()
          }
        }
      }
      event "停止应用程序 3": Value Change {
        n207 = event-data() -> ()  [unwired: 1 in, 6 out]
        n208 = Not(x="停止应用程序 3") -> (.not. x?=w517:bool)
        n209 = shared-variable "roboRIO-1256-FRC\\Shared Variable.lvlib\\Active"(w517, error in=w516) -> (error out=w515:errorcluster)
      }
    }
  }
  n210 = while {
    tunnel: w106 -> [w526]
    tunnel: [w521] -> w101
    tunnel: w105 -> [w525]
    tunnel: [w523] -> w103
    tunnel: w104 -> [w524]
    tunnel: [w522] -> w102
    stop <- FALSE stop-if-true
    n211 = event shown="[0] Timeout" {
      selector: _ -> [_ _]
      dyn-events: _ -> [_ _]
      timeout: 250 -> [_ _]
      tunnel: w524 -> [w532 w562]
      tunnel: [w535 w561] -> w522
      tunnel: w525 -> [w531 w559]
      tunnel: [w534 w559] -> w523
      tunnel: w526 -> [w533 w560]
      tunnel: [w533 w560] -> w521
      event Timeout {
        n212 = event-data() -> ()  [unwired: 1 in, 3 out]
        n213 = property class="Network Stream Endpoint"(reference=w531, error in=w532) -> (reference out=w529:refnum<k21>, error out=w530:errorcluster, "AvailElmntsForRead"=w528:i32)
        n214 = Greater Than 0?(x=w528) -> (x > 0?=w527:bool)
        n215 = case shown="True" w527 {
          tunnel: [w536 w551] -> w535
          tunnel: [w537 w550] -> w534
          tunnel: w533 -> [_ w543]
          tunnel: w530 -> [w536 w545]
          tunnel: w529 -> [w537 w544]
          frame False {
          }
          frame True {
            n216 = shared-variable-read(w544, w545) -> (w550:refnum<k21>, w551:errorcluster, w541:i32[])  [unwired: 1 in, 1 out]
            n217 = shared-variable "roboRIO-1256-FRC\\Shared Variable.lvlib\\Height"() -> (w538:u16)  [unwired: 1 in, 1 out]
            n218 = feedback #9() -> (w539:i32[][])  [unwired: 1 in]
            n219 = Build Array (concatenate)(w539, w541) -> (w542:i32[][])
            n220 = Index Array(array=w542, index (col)=0 ("disabled index (col)")) -> (element=w548:i32[])  [unwired: 1 in]
            n221 = Array Size(array=w548) -> (size(s)=w547:i32)
            n222 = Equal?(x=w547, y=w538) -> (x = y?=w546:bool)
            n223 = case shown="True" w546 {
              tunnel: w542 -> [w552 w553]
              tunnel: [w552 w554] -> w540
              tunnel: w538 -> [_ w558]
              tunnel: w543 -> [_ w555]
              frame False {
              }
              frame True {
                n224 = Delete From Array(array=w553, length=w558, index (row)=0) -> (array with subset deleted=w554:i32[][])  [unwired: 1 in, 1 out]
                n225 = call "IMAQ ArrayToImage"("Image Pixels (U8)"=w553, "Image"=w555) -> ("Image Out"=→"Gaussian1-3":T1)  [unwired: 8 in, 1 out]
                "Array 3" <- w553
              }
            }
            n226 = feedback-in #9(w540) -> ()
          }
        }
      }
      event "停止应用程序 3": Value Change {
        n227 = event-data() -> ()  [unwired: 1 in, 6 out]
        n228 = Not(x="停止应用程序 4") -> (.not. x?=w563:bool)
        n229 = shared-variable "roboRIO-1256-FRC\\Shared Variable.lvlib\\Active"(w563, error in=w562) -> (error out=w561:errorcluster)
      }
    }
  }
  n230 = while {
    tunnel: w112 -> [w572]
    tunnel: [w567] -> w107
    tunnel: w111 -> [w571]
    tunnel: [w568] -> w108
    tunnel: w110 -> [w570]
    tunnel: [w569] -> w109
    stop <- FALSE stop-if-true
    n231 = event shown="[0] Timeout" {
      selector: _ -> [_ _]
      dyn-events: _ -> [_ _]
      timeout: 250 -> [_ _]
      tunnel: w570 -> [w578 w608]
      tunnel: [w581 w607] -> w569
      tunnel: w571 -> [w577 w605]
      tunnel: [w580 w605] -> w568
      tunnel: w572 -> [w579 w606]
      tunnel: [w579 w606] -> w567
      event Timeout {
        n232 = event-data() -> ()  [unwired: 1 in, 3 out]
        n233 = property class="Network Stream Endpoint"(reference=w577, error in=w578) -> (reference out=w575:refnum<k21>, error out=w576:errorcluster, "AvailElmntsForRead"=w574:i32)
        n234 = Greater Than 0?(x=w574) -> (x > 0?=w573:bool)
        n235 = case shown="True" w573 {
          tunnel: [w582 w597] -> w581
          tunnel: [w583 w596] -> w580
          tunnel: w579 -> [_ w589]
          tunnel: w576 -> [w582 w591]
          tunnel: w575 -> [w583 w590]
          frame False {
          }
          frame True {
            n236 = shared-variable-read(w590, w591) -> (w596:refnum<k21>, w597:errorcluster, w587:i32[])  [unwired: 1 in, 1 out]
            n237 = shared-variable "roboRIO-1256-FRC\\Shared Variable.lvlib\\Height"() -> (w584:u16)  [unwired: 1 in, 1 out]
            n238 = feedback #10() -> (w585:i32[][])  [unwired: 1 in]
            n239 = Build Array (concatenate)(w585, w587) -> (w588:i32[][])
            n240 = Index Array(array=w588, index (col)=0 ("disabled index (col)")) -> (element=w594:i32[])  [unwired: 1 in]
            n241 = Array Size(array=w594) -> (size(s)=w593:i32)
            n242 = Equal?(x=w593, y=w584) -> (x = y?=w592:bool)
            n243 = case shown="True" w592 {
              tunnel: w588 -> [w598 w599]
              tunnel: [w598 w600] -> w586
              tunnel: w584 -> [_ w604]
              tunnel: w589 -> [_ w601]
              frame False {
              }
              frame True {
                n244 = Delete From Array(array=w599, length=w604, index (row)=0) -> (array with subset deleted=w600:i32[][])  [unwired: 1 in, 1 out]
                n245 = call "IMAQ ArrayToImage"("Image Pixels (U8)"=w599, "Image"=w601) -> ("Image Out"=→"Gaussian1-4":T1)  [unwired: 8 in, 1 out]
                "Array 4" <- w599
              }
            }
            n246 = feedback-in #10(w586) -> ()
          }
        }
      }
      event "停止应用程序 3": Value Change {
        n247 = event-data() -> ()  [unwired: 1 in, 6 out]
        n248 = Not(x="停止应用程序 5") -> (.not. x?=w609:bool)
        n249 = shared-variable "roboRIO-1256-FRC\\Shared Variable.lvlib\\Active"(w609, error in=w608) -> (error out=w607:errorcluster)
      }
    }
  }
  n250 = while {
    tunnel: w77 -> [w618]
    tunnel: [w613] -> w72
    tunnel: w76 -> [w617]
    tunnel: [w614] -> w73
    tunnel: w75 -> [w616]
    tunnel: [w615] -> w74
    stop <- FALSE stop-if-true
    n251 = event shown="[0] Timeout" {
      selector: _ -> [_ _]
      dyn-events: _ -> [_ _]
      timeout: 250 -> [_ _]
      tunnel: w616 -> [w624 w654]
      tunnel: [w627 w653] -> w615
      tunnel: w617 -> [w623 w651]
      tunnel: [w626 w651] -> w614
      tunnel: w618 -> [w625 w652]
      tunnel: [w625 w652] -> w613
      event Timeout {
        n252 = event-data() -> ()  [unwired: 1 in, 3 out]
        n253 = property class="Network Stream Endpoint"(reference=w623, error in=w624) -> (reference out=w621:refnum<k21>, error out=w622:errorcluster, "AvailElmntsForRead"=w620:i32)
        n254 = Greater Than 0?(x=w620) -> (x > 0?=w619:bool)
        n255 = case shown="True" w619 {
          tunnel: [w628 w643] -> w627
          tunnel: [w629 w642] -> w626
          tunnel: w625 -> [_ w635]
          tunnel: w622 -> [w628 w637]
          tunnel: w621 -> [w629 w636]
          frame False {
          }
          frame True {
            n256 = shared-variable-read(w636, w637) -> (w642:refnum<k21>, w643:errorcluster, w633:i32[])  [unwired: 1 in, 1 out]
            n257 = shared-variable "roboRIO-1256-FRC\\Shared Variable.lvlib\\deHeight"() -> (w630:u16)  [unwired: 1 in, 1 out]
            n258 = feedback #11() -> (w631:i32[][])  [unwired: 1 in]
            n259 = Build Array (concatenate)(w631, w633) -> (w634:i32[][])
            n260 = Index Array(array=w634, index (col)=0 ("disabled index (col)")) -> (element=w640:i32[])  [unwired: 1 in]
            n261 = Array Size(array=w640) -> (size(s)=w639:i32)
            n262 = Equal?(x=w639, y=w630) -> (x = y?=w638:bool)
            n263 = case shown="True" w638 {
              tunnel: w634 -> [w644 w645]
              tunnel: [w644 w646] -> w632
              tunnel: w630 -> [_ w650]
              tunnel: w635 -> [_ w647]
              frame False {
              }
              frame True {
                n264 = Delete From Array(array=w645, length=w650, index (row)=0) -> (array with subset deleted=w646:i32[][])  [unwired: 1 in, 1 out]
                n265 = call "IMAQ ArrayToImage"("Image Pixels (U8)"=w645, "Image"=w647) -> ("Image Out"=→"Gaussian2-2":T1)  [unwired: 8 in, 1 out]
                "Array 6" <- w645
              }
            }
            n266 = feedback-in #11(w632) -> ()
          }
        }
      }
      event "停止应用程序 3": Value Change {
        n267 = event-data() -> ()  [unwired: 1 in, 6 out]
        n268 = Not(x="停止应用程序 7") -> (.not. x?=w655:bool)
        n269 = shared-variable "roboRIO-1256-FRC\\Shared Variable.lvlib\\Active"(w655, error in=w654) -> (error out=w653:errorcluster)
      }
    }
  }
  n270 = while {
    tunnel: w66 -> [w664]
    tunnel: [w659] -> w71
    tunnel: w67 -> [w663]
    tunnel: [w660] -> w70
    tunnel: w68 -> [w662]
    tunnel: [w661] -> w69
    stop <- FALSE stop-if-true
    n271 = event shown="[0] Timeout" {
      selector: _ -> [_ _]
      dyn-events: _ -> [_ _]
      timeout: 250 -> [_ _]
      tunnel: w662 -> [w670 w700]
      tunnel: [w673 w699] -> w661
      tunnel: w663 -> [w669 w697]
      tunnel: [w672 w697] -> w660
      tunnel: w664 -> [w671 w698]
      tunnel: [w671 w698] -> w659
      event Timeout {
        n272 = event-data() -> ()  [unwired: 1 in, 3 out]
        n273 = property class="Network Stream Endpoint"(reference=w669, error in=w670) -> (reference out=w667:refnum<k21>, error out=w668:errorcluster, "AvailElmntsForRead"=w666:i32)
        n274 = Greater Than 0?(x=w666) -> (x > 0?=w665:bool)
        n275 = case shown="True" w665 {
          tunnel: [w674 w689] -> w673
          tunnel: [w675 w688] -> w672
          tunnel: w671 -> [_ w681]
          tunnel: w668 -> [w674 w683]
          tunnel: w667 -> [w675 w682]
          frame False {
          }
          frame True {
            n276 = shared-variable-read(w682, w683) -> (w688:refnum<k21>, w689:errorcluster, w679:i32[])  [unwired: 1 in, 1 out]
            n277 = shared-variable "roboRIO-1256-FRC\\Shared Variable.lvlib\\deHeight"() -> (w676:u16)  [unwired: 1 in, 1 out]
            n278 = feedback #12() -> (w677:i32[][])  [unwired: 1 in]
            n279 = Build Array (concatenate)(w677, w679) -> (w680:i32[][])
            n280 = Index Array(array=w680, index (col)=0 ("disabled index (col)")) -> (element=w686:i32[])  [unwired: 1 in]
            n281 = Array Size(array=w686) -> (size(s)=w685:i32)
            n282 = Equal?(x=w685, y=w676) -> (x = y?=w684:bool)
            n283 = case shown="True" w684 {
              tunnel: w680 -> [w690 w691]
              tunnel: [w690 w692] -> w678
              tunnel: w676 -> [_ w696]
              tunnel: w681 -> [_ w693]
              frame False {
              }
              frame True {
                n284 = Delete From Array(array=w691, length=w696, index (row)=0) -> (array with subset deleted=w692:i32[][])  [unwired: 1 in, 1 out]
                n285 = call "IMAQ ArrayToImage"("Image Pixels (U8)"=w691, "Image"=w693) -> ("Image Out"=→"Gaussian2-3":T1)  [unwired: 8 in, 1 out]
                "Array 7" <- w691
              }
            }
            n286 = feedback-in #12(w678) -> ()
          }
        }
      }
      event "停止应用程序 3": Value Change {
        n287 = event-data() -> ()  [unwired: 1 in, 6 out]
        n288 = Not(x="停止应用程序 8") -> (.not. x?=w701:bool)
        n289 = shared-variable "roboRIO-1256-FRC\\Shared Variable.lvlib\\Active"(w701, error in=w700) -> (error out=w699:errorcluster)
      }
    }
  }
  n290 = while {
    tunnel: w43 -> [w708]
    tunnel: [w705] -> w46
    tunnel: w44 -> [w707]
    tunnel: [w706] -> w45
    stop <- FALSE stop-if-true
    n291 = event shown="[0] Timeout" {
      selector: _ -> [_ _]
      dyn-events: _ -> [_ _]
      timeout: 250 -> [_ _]
      tunnel: w707 -> [w714 w739]
      tunnel: [w716 w738] -> w706
      tunnel: w708 -> [w713 w737]
      tunnel: [w715 w737] -> w705
      event Timeout {
        n292 = event-data() -> ()  [unwired: 1 in, 3 out]
        n293 = property class="Network Stream Endpoint"(reference=w713, error in=w714) -> (reference out=w711:refnum<k21>, error out=w712:errorcluster, "AvailElmntsForRead"=w710:i32)
        n294 = Greater Than 0?(x=w710) -> (x > 0?=w709:bool)
        n295 = case shown="True" w709 {
          tunnel: [w717 w731] -> w716
          tunnel: [w718 w730] -> w715
          tunnel: w712 -> [w717 w725]
          tunnel: w711 -> [w718 w724]
          frame False {
          }
          frame True {
            n296 = shared-variable-read(w724, w725) -> (w730:refnum<k21>, w731:errorcluster, w722:i32[])  [unwired: 1 in, 1 out]
            n297 = shared-variable "roboRIO-1256-FRC\\Shared Variable.lvlib\\Height"() -> (w719:u16)  [unwired: 1 in, 1 out]
            n298 = feedback #13() -> (w720:i32[][])  [unwired: 1 in]
            n299 = Build Array (concatenate)(w720, w722) -> (w723:i32[][])
            n300 = Index Array(array=w723, index (col)=0 ("disabled index (col)")) -> (element=w728:i32[])  [unwired: 1 in]
            n301 = Array Size(array=w728) -> (size(s)=w727:i32)
            n302 = Equal?(x=w727, y=w719) -> (x = y?=w726:bool)
            n303 = case shown="True" w726 {
              tunnel: w723 -> [w732 w733]
              tunnel: [w732 w734] -> w721
              tunnel: w719 -> [_ w736]
              frame False {
              }
              frame True {
                n304 = Delete From Array(array=w733, length=w736, index (row)=0) -> (array with subset deleted=w734:i32[][])  [unwired: 1 in, 1 out]
                "Array 9" <- w733
              }
            }
            n305 = feedback-in #13(w721) -> ()
          }
        }
      }
      event "停止应用程序 3": Value Change {
        n306 = event-data() -> ()  [unwired: 1 in, 6 out]
        n307 = Not(x="停止应用程序 10") -> (.not. x?=w740:bool)
        n308 = shared-variable "roboRIO-1256-FRC\\Shared Variable.lvlib\\Active"(w740, error in=w739) -> (error out=w738:errorcluster)
      }
    }
  }
  n309 = while {
    tunnel: w89 -> [w749]
    tunnel: [w744] -> w94
    tunnel: w90 -> [w748]
    tunnel: [w745] -> w93
    tunnel: w91 -> [w747]
    tunnel: [w746] -> w92
    stop <- FALSE stop-if-true
    n310 = event shown="[0] Timeout" {
      selector: _ -> [_ _]
      dyn-events: _ -> [_ _]
      timeout: 250 -> [_ _]
      tunnel: w747 -> [w755 w785]
      tunnel: [w758 w784] -> w746
      tunnel: w748 -> [w754 w782]
      tunnel: [w757 w782] -> w745
      tunnel: w749 -> [w756 w783]
      tunnel: [w756 w783] -> w744
      event Timeout {
        n311 = event-data() -> ()  [unwired: 1 in, 3 out]
        n312 = property class="Network Stream Endpoint"(reference=w754, error in=w755) -> (reference out=w752:refnum<k21>, error out=w753:errorcluster, "AvailElmntsForRead"=w751:i32)
        n313 = Greater Than 0?(x=w751) -> (x > 0?=w750:bool)
        n314 = case shown="True" w750 {
          tunnel: [w759 w774] -> w758
          tunnel: [w760 w773] -> w757
          tunnel: w756 -> [_ w766]
          tunnel: w753 -> [w759 w768]
          tunnel: w752 -> [w760 w767]
          frame False {
          }
          frame True {
            n315 = shared-variable-read(w767, w768) -> (w773:refnum<k21>, w774:errorcluster, w764:i32[])  [unwired: 1 in, 1 out]
            n316 = shared-variable "roboRIO-1256-FRC\\Shared Variable.lvlib\\deHeight"() -> (w761:u16)  [unwired: 1 in, 1 out]
            n317 = feedback #14() -> (w762:i32[][])  [unwired: 1 in]
            n318 = Build Array (concatenate)(w762, w764) -> (w765:i32[][])
            n319 = Index Array(array=w765, index (col)=0 ("disabled index (col)")) -> (element=w771:i32[])  [unwired: 1 in]
            n320 = Array Size(array=w771) -> (size(s)=w770:i32)
            n321 = Equal?(x=w770, y=w761) -> (x = y?=w769:bool)
            n322 = case shown="True" w769 {
              tunnel: w765 -> [w775 w776]
              tunnel: [w775 w777] -> w763
              tunnel: w761 -> [_ w781]
              tunnel: w766 -> [_ w778]
              frame False {
              }
              frame True {
                n323 = Delete From Array(array=w776, length=w781, index (row)=0) -> (array with subset deleted=w777:i32[][])  [unwired: 1 in, 1 out]
                n324 = call "IMAQ ArrayToImage"("Image Pixels (U8)"=w776, "Image"=w778) -> ("Image Out"=→"Gaussian2-1":T1)  [unwired: 8 in, 1 out]
                "Array 5" <- w776
              }
            }
            n325 = feedback-in #14(w763) -> ()
          }
        }
      }
      event "停止应用程序 3": Value Change {
        n326 = event-data() -> ()  [unwired: 1 in, 6 out]
        n327 = Not(x="停止应用程序 6") -> (.not. x?=w786:bool)
        n328 = shared-variable "roboRIO-1256-FRC\\Shared Variable.lvlib\\Active"(w786, error in=w785) -> (error out=w784:errorcluster)
      }
    }
  }
  n329 = call "IMAQ Dispose"("Image"=w134) -> ()  [unwired: 5 in, 1 out]
  n330 = Destroy Stream Endpoint(8:w141, 11:w139) -> (0:→"error out 2":errorcluster)
  n331 = Destroy Stream Endpoint(8:w6, 11:w5) -> ()  [unwired: 1 out]
  n332 = Destroy Stream Endpoint(8:w20, 11:w19) -> ()  [unwired: 1 out]
  n333 = Destroy Stream Endpoint(8:w17, 11:w18) -> ()  [unwired: 1 out]
  n334 = Destroy Stream Endpoint(8:w95, 11:w96) -> (0:w120:errorcluster)
  n335 = call "IMAQ Dispose"("Image"=w101) -> ()  [unwired: 5 in, 1 out]
  n336 = Destroy Stream Endpoint(8:w102, 11:w103) -> (0:w119:errorcluster)
  n337 = Destroy Stream Endpoint(8:w31, 11:w32) -> ()  [unwired: 1 out]
  n338 = Destroy Stream Endpoint(8:w151, 11:w150) -> (0:w121:errorcluster)
  n339 = call "IMAQ Dispose"("Image"=w97) -> ()  [unwired: 5 in, 1 out]
  n340 = Destroy Stream Endpoint(8:w34, 11:w33) -> ()  [unwired: 1 out]
  n341 = call "IMAQ Dispose"("Image"=w50) -> ()  [unwired: 5 in, 1 out]
  n342 = Destroy Stream Endpoint(8:w52, 11:w51) -> (0:w47:errorcluster)
  n343 = call "IMAQ Dispose"("Image"=w107) -> ()  [unwired: 5 in, 1 out]
  n344 = Destroy Stream Endpoint(8:w109, 11:w108) -> (0:w113:errorcluster)
  n345 = call "IMAQ Dispose"("Image"=w72) -> ()  [unwired: 5 in, 1 out]
  n346 = Destroy Stream Endpoint(8:w74, 11:w73) -> (0:w49:errorcluster)
  n347 = call "IMAQ Dispose"("Image"=w71) -> ()  [unwired: 5 in, 1 out]
  n348 = Destroy Stream Endpoint(8:w69, 11:w70) -> (0:w48:errorcluster)
  n349 = Destroy Stream Endpoint(8:w45, 11:w46) -> ()  [unwired: 1 out]
  n350 = call "IMAQ Dispose"("Image"=w94) -> ()  [unwired: 5 in, 1 out]
  n351 = Destroy Stream Endpoint(8:w92, 11:w93) -> (0:w83:errorcluster)
  n352 = call "IMAQ Dispose"("Image"=w147) -> ()  [unwired: 5 in, 1 out]
  n353 = Merge Errors(w121, w120, w119, w113, w83, w49, w48, w47) -> (→"error out":errorcluster)
